vi "Read Active Time Entry GUID.vi"(8 "error in (no error)":errorcluster, 11 "Time Entries in":refnum<class "Time Entries.lvclass">) -> (0 "error out":errorcluster, 2 "Active Time Entry GUID":string, 3 "Time Entries out":refnum<class "Time Entries.lvclass">)   [LabVIEW 2020, in "Time Entries.lvclass"]
uses:
  Time Entries.lvclass
  Time Entries.lvclass/Time Entries.ctl
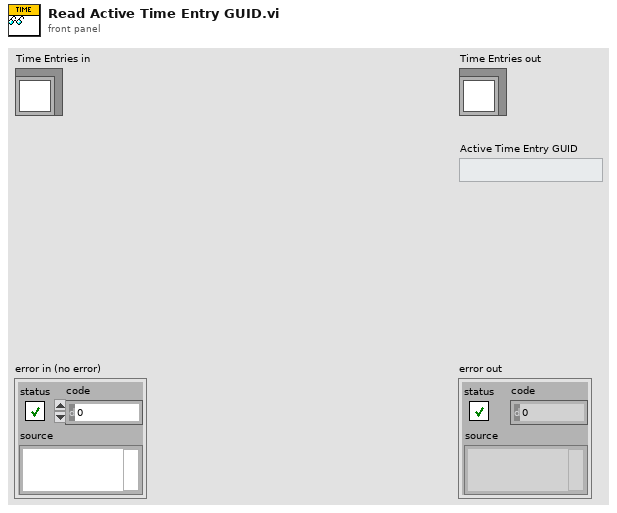
[diagram p1: front panel]
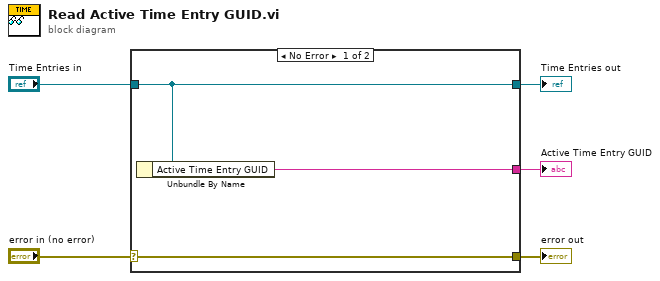
[diagram p0: block diagram]
diagram:
  n1 = case shown="No Error" "error in (no error)" {
    selector: "error in (no error)" -> [w8 w9]
    tunnel: [w8 w9] -> w4
    tunnel: [w7 w10] -> w2
    tunnel: "Time Entries in" -> [w7 w10]
    tunnel: [w6 _] -> w1
    frame No Error {
      n2 = Unbundle By Name(w7) -> ("Active Time Entry GUID"=w6:string)
    }
    frame Error {
    }
  }
  "error out" <- w4
  "Time Entries out" <- w2
  "Active Time Entry GUID" <- w1
